vi "mbug_2820_select.vi"() -> ()   [LabVIEW 2014]
doc: "This example shows how to acquire a power measurement using the VIs of the driver."
uses:
  <instrlib>/MBUG-2820/Private/Open_id.vi
  <instrlib>/MBUG-2820/MBUG-2820.lvlib
panel:
  in  "Select device":string(combo)
  out "Rel. humidity (%)":dbl
  out "Temperature (°C)":dbl
  # "MBUG-2820 select device example"
  # "Choose a device from\nthe Combobox to take\na single measurement."
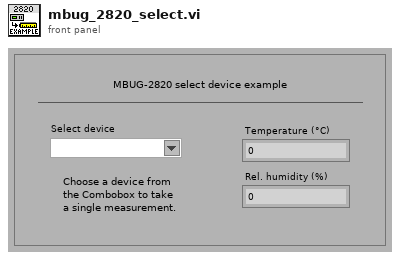
[diagram p1: front panel]
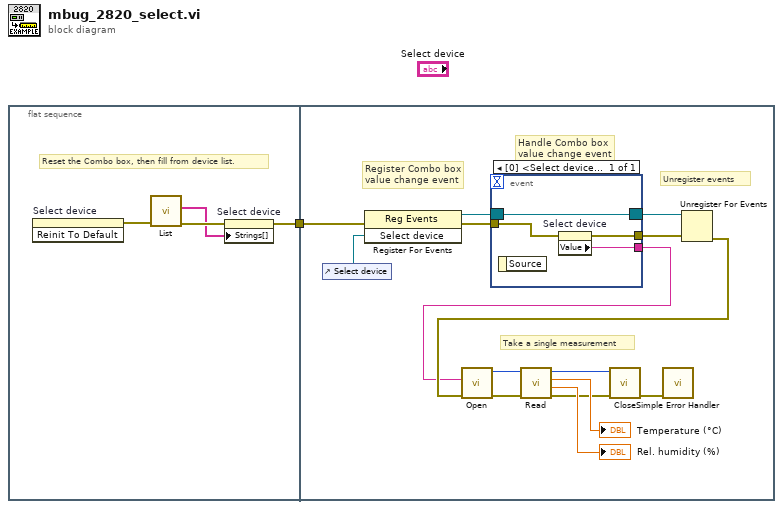
[diagram p0: block diagram]
diagram:
  n1 = flat-sequence {
    tunnel: [w3] -> w1
    tunnel: w1 -> [w10]
    frame #0 {
      # "Reset the Combo box, then fill from device list."
      n2 = invoke on="Select device" class="CmbBox" method="Reinit To Default"() -> (error out=w5:errorcluster)  [unwired: 3 in, 2 out]
      n3 = call <instrlib>:"List.vi"("error in (no error)"=w5) -> ("error out"=w4:errorcluster, "Device id strings"=w2:string[])  [unwired: 4 in, 1 out]
      n4 = property on="Select device" class="CmbBox"(error in=w4, "Strings[]"=w2) -> (error out=w3:errorcluster)  [unwired: 1 in, 1 out]
    }
    frame #1 {
      # "Take a single measurement"
      # "Unregister events"
      # "Handle Combo box\nvalue change event"
      # "Register Combo box\nvalue change event"
      n5 = control-ref of="Select device"() -> (w11:refnum<vi>)
      n6 = register-events(error in=w10, w11) -> (reference out=w12:refnum<event-registration>, error out=w15:errorcluster)  [unwired: 1 in]
      n7 = event shown="[0] <Select device>: Value Change" {
        selector: w12 -> [w24]
        dyn-events: [w24] -> w13
        timeout: _ -> [_]
        tunnel: [w22] -> w14
        tunnel: w15 -> [w23]
        tunnel: [w21] -> w6
        event Value Change {
          n8 = event-data() -> ()  [unwired: 1 in, 1 out]
          n9 = property on="Select device" class="CmbBox"(error in=w23) -> (error out=w22:errorcluster, "Value"=w21:string)  [unwired: 1 in, 1 out]
        }
      }
      n10 = Unregister For Events(event registration refnum=w13, error in=w14) -> (error out=w7:errorcluster)
      n11 = call-poly <instrlib>:"Open.vi"("error in (no error)"=w7, "Device id string"=w6) -> ("error out"=w8:errorcluster, "Device handle"=w9:u32)  [unwired: 4 in]
      n12 = call <instrlib>:"Read.vi"("error in (no error)"=w8, "Device handle in"=w9) -> ("error out"=w17:errorcluster, "Rel. humidity (%)"=→"Rel. humidity (%)":dbl, "Temperature (°C)"=→"Temperature (°C)":dbl, "Device handle out"=w16:u32)  [unwired: 2 in]
      n13 = call <instrlib>:"Close.vi"("error in (no error)"=w17, "Device handle"=w16) -> ("error out"=w18:errorcluster)  [unwired: 5 in]
      n14 = call <vilib>:"Simple Error Handler.vi"("error in (no error)"=w18) -> ()  [unwired: 4 in, 5 out]
    }
  }
